vi "BL Calc Peak Find.vi"(4 "back emf":dbl[](array[numeric]), 6 "cap probe":dbl[](array[numeric]), 8 "threshold valleys":dbl, 9 "threshold peaks":dbl, 10 "width":i32, 11 "frequency (Hz)":dbl) -> (3 "Numeric":dbl)   [LabVIEW 2018]
uses:
  <vilib>/Analysis/baseanly.llb/Mean (DBL).vi
  <vilib>/Analysis/NI_AAL_SigProc.lvlib
  <vilib>/Analysis/NI_AALBase.lvlib
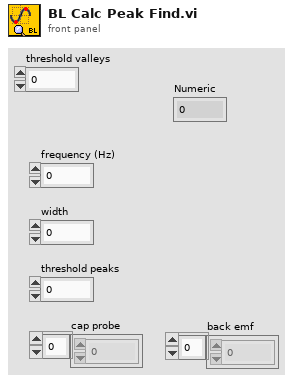
[diagram p1: front panel]
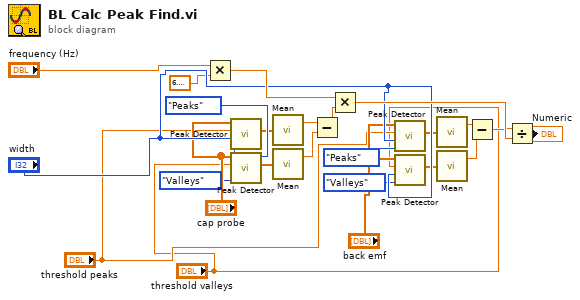
[diagram p0: block diagram]
diagram:
  n1 = Multiply(x="frequency (Hz)", y=6.283185307179586) -> (x*y=w24:dbl)
  n2 = call <vilib>:"Peak Detector.vi"("peaks/valleys"=enum32{"Peaks", "Valleys"}."Peaks", "width"="width", "threshold"="threshold peaks", "X"="cap probe") -> ("Amplitudes"=w3:dbl[])  [unwired: 3 in, 4 out]
  n3 = call <vilib>:"Peak Detector.vi"("peaks/valleys"=enum32{"Peaks", "Valleys"}."Valleys", "threshold"="threshold valleys", "X"="cap probe") -> ("Amplitudes"=w6:dbl[])  [unwired: 4 in, 4 out]
  n4 = call-poly <vilib>:"Mean.vi"("X"=w3) -> ("mean"=w22:dbl)  [unwired: 1 out]
  n5 = call-poly <vilib>:"Mean.vi"("X"=w6) -> ("mean"=w23:dbl)  [unwired: 1 out]
  n6 = Subtract(x=w22, y=w23) -> (x-y=w17:dbl)
  n7 = Multiply(x=w24, y=w17) -> (x*y=w21:dbl)
  n8 = call <vilib>:"Peak Detector.vi"("peaks/valleys"=enum32{"Peaks", "Valleys"}."Peaks", "width"="width", "threshold"="threshold peaks", "X"="back emf") -> ("Amplitudes"=w7:dbl[])  [unwired: 3 in, 4 out]
  n9 = call <vilib>:"Peak Detector.vi"("peaks/valleys"=enum32{"Peaks", "Valleys"}."Valleys", "width"="width", "threshold"="threshold valleys", "X"="back emf") -> ("Amplitudes"=w8:dbl[])  [unwired: 3 in, 4 out]
  n10 = call-poly <vilib>:"Mean.vi"("X"=w7) -> ("mean"=w9:dbl)  [unwired: 1 out]
  n11 = call-poly <vilib>:"Mean.vi"("X"=w8) -> ("mean"=w10:dbl)  [unwired: 1 out]
  n12 = Subtract(x=w9, y=w10) -> (x-y=w20:dbl)
  n13 = Divide(x=w20, y=w21) -> (x/y=→"Numeric":dbl)
